vi "Flush.vi"(11 "TypedCircularBuffer in":refnum<class "RotateCircularBuffer.lvclass">) -> (2 "Array":T1[](array[typedef]), 3 "TypedCircularBuffer out":refnum<class "RotateCircularBuffer.lvclass">)   [LabVIEW 2024, in "RotateCircularBuffer.lvclass"]
uses:
  RotateCircularBuffer.lvclass
  Type.ctl
  RotateCircularBuffer.lvclass/RotateCircularBuffer.ctl
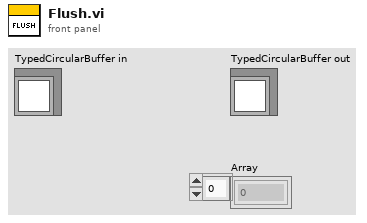
[diagram p1: front panel]
types:
  T1 = typedef "RotateCircularBuffer.lvclass/Type.ctl" = u8
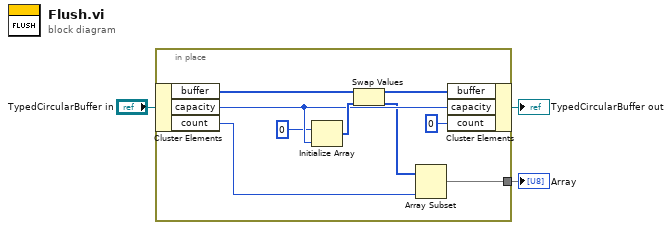
[diagram p0: block diagram]
diagram:
  n1 = in-place {
    in-place-border: [w4] -> w1
    n2 = in-place-cluster #1("TypedCircularBuffer in") -> ("buffer"=w12:T1[], "capacity"=w9:u32, "count"=w5:u32)
    n3 = Initialize Array(T1 0 ("Type"), w9) -> (w11:T1[])
    n4 = Swap Values(12:w12, 14:w11) -> (1:w10:T1[], 3:w6:T1[])  [unwired: 1 in]
    n5 = Array Subset(array=w6, length=w5) -> (w4:T1[])  [unwired: 1 in]
    n6 = in-place-cluster #1("buffer"=w10, "capacity"=w9, "count"=u32 0 ("head")) -> (→"TypedCircularBuffer out":refnum<class "RotateCircularBuffer.lvclass">)
  }
  "Array" <- w1
